vi "Save Settings to XML.vi"(8 "error in (no error)":errorcluster caption="错误输入（无错误）", 11 "Settings":T1 caption="设置") -> (0 "error out":errorcluster caption="错误输出")   [LabVIEW 2015, in "Settings.lvlib"]
doc: "将用户设定的配置数据保存至XML文件。本VI可在多次执行之间保持用户设置。"
uses:
  Settings.lvlib
  <vilib>/Utility/xml.llb/Write to XML File(string).vi
  Acquisition/Hardware Configuration.ctl
  Logging/Logging Configuration.ctl
  Settings.ctl
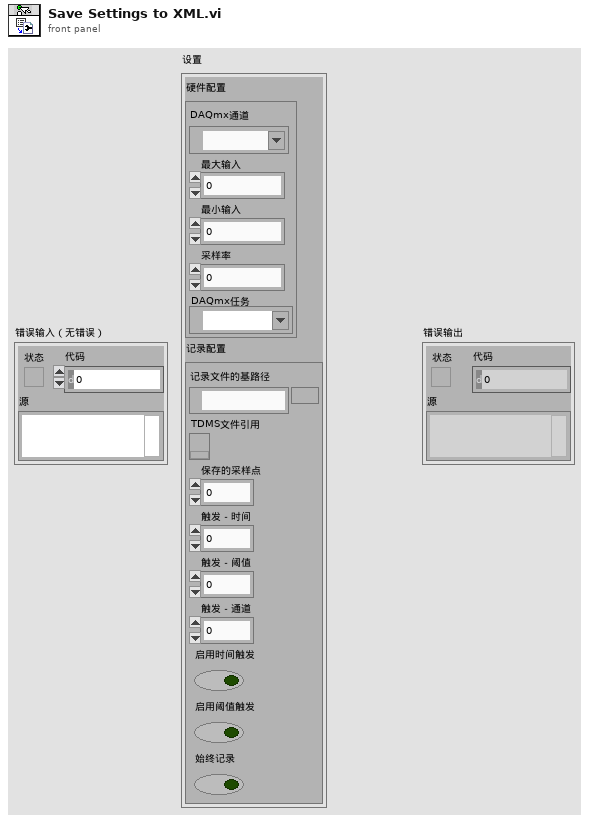
[diagram p1: front panel]
types:
  T1 = typedef "Settings.lvlib/Settings.ctl" = cluster{"Hardware Configuration":T2, "Logging Configuration":T3}
  T2 = typedef "Acquisition.lvlib/Hardware Configuration.ctl" = cluster{"DAQmx Channel":tag, "Max Input":dbl, "Min Input":dbl, "Sample Rate":dbl, "DAQmx Task":refnum<k21>}
  T3 = typedef "Logging.lvlib/Logging Configuration.ctl" = cluster{"Log File Base Path":path, "TDMS File Reference":refnum<k34>, "Samples to Save":u32, "Trigger - Time":u32, "Trigger - Threshold":dbl, "Trigger - Channel":u32, "Enable Time Trigger":bool, "Enable Threshold Trigger":bool, "Always Log":bool}
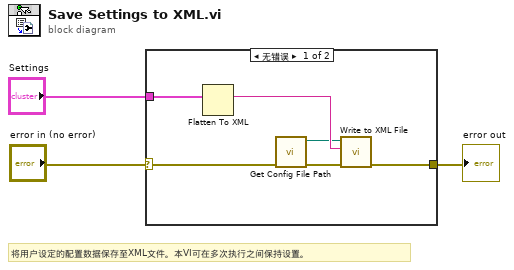
[diagram p0: block diagram]
diagram:
  # "将用户设定的配置数据保存至XML文件。本VI可在多次执行之间保持设置。"
  n1 = case shown="无错误" "error in (no error)" {
    selector: "error in (no error)" -> [w5 w10]
    tunnel: [w7 w10] -> w2
    tunnel: "Settings" -> [w9 _]
    frame No Error {
      n2 = Flatten To XML(anything=w9) -> (xml string=w8:string)
      n3 = call "Get Config File Path.vi"("error in (no error)"=w5) -> ("error out"=w4:errorcluster, "XML File Path"=w6:path)  [unwired: 9 in]
      n4 = call-poly <vilib>:"Write to XML File.vi"("error in (no error)"=w4, "XML Input"=w8, "XML File Path"=w6) -> ("error out"=w7:errorcluster)  [unwired: 6 in, 2 out]
    }
    frame Error {
    }
  }
  "error out" <- w2
